vi "NapovedaEEG(subVI).vi"() -> ()   [LabVIEW 2026]
panel:
  in  "Close":bool
  # "1. Místa na hlavě (pokožku), kam budete umisťovat elektrody, je nutné řádně očistit. \n    Pokud jsou v místě vlasy, snažte se je rozhrnout. U EEG je klíčový dobrý kontakt.\n2. Vybalte a nalepte na dobrovolníka elektrody. Typicky se používá umístění na čele (Fp1/Fp2) a za uchem nebo na týlu.\n3. Označení elektrod je na PLUX BITalino následující:\n      - černá a červená: aktivní elektrody (nalepte na místa měřené aktivity, např. na levé a pravé čelo).\n      - bílá: referenční elektroda (nalepte na kost za uchem – mastoid – nebo na ušní lalůček).\n4. Na nalepené elektrody nacvakněte kabely od PLUX BITalina.\n5. Kabel s elektrodami připojte do propojky s nápisem EEG do portu, u kterého není nápis EEG.\n6. Do propojky k nápisu EEG zapojte propojovací kabel a jeho druhý konec do portu A2 (nebo dle instrukcí k úloze).\n7. Zapněte PLUX BITalino (LED musí pulsovat).\n8. EEG signál je velmi slabý (uV), proto se snažte, aby byl dobrovolník v klidu a nemrkal."
  # "Zapojení elektrod do bílé propojky s filtry a zesilovači"
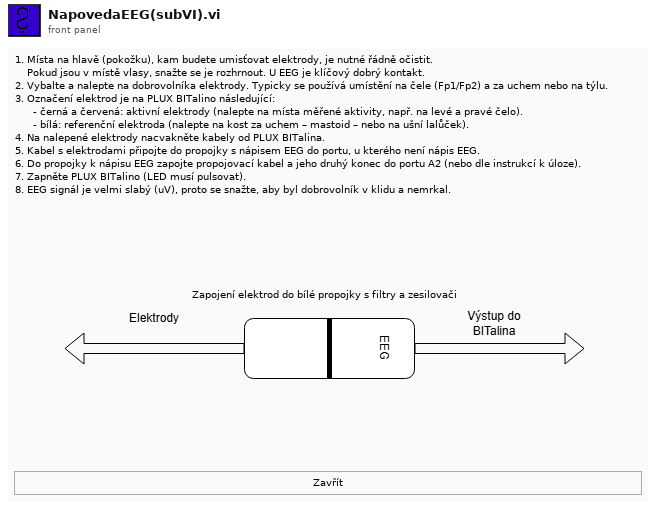
[diagram p1: front panel]
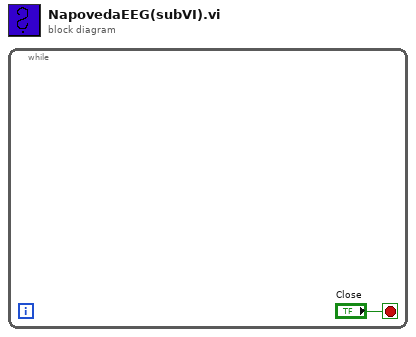
[diagram p0: block diagram]
diagram:
  n1 = while {
    stop <- "Close" stop-if-true
  }
